vi "pruebas con Alarm Log.vi"() -> ()   [LabVIEW 2018]
panel:
  out "Array":i16[][](array[numeric])
  in  "Descending (F)":bool
  out "PQ_Log array out 4":i16[][](array[numeric])
  out "Numeric":i32
  out "PQ_Log array out":i16[](array[numeric])
  out "Boolean array 6":bool[](array[boolean])
  in  "stop":bool
  # "Sag_Indication_Detected"
  # "Swell_Indication_Detected"
  # "Transient_Indication"
  # "200mS_Sag_Swell_Status_Flag"
  # "3s_Sag_Swell_Status_Flag"
  # "10m_Sag_Swell_Status_Flag"
  # "2h_Sag_Swell_Status_Flag"
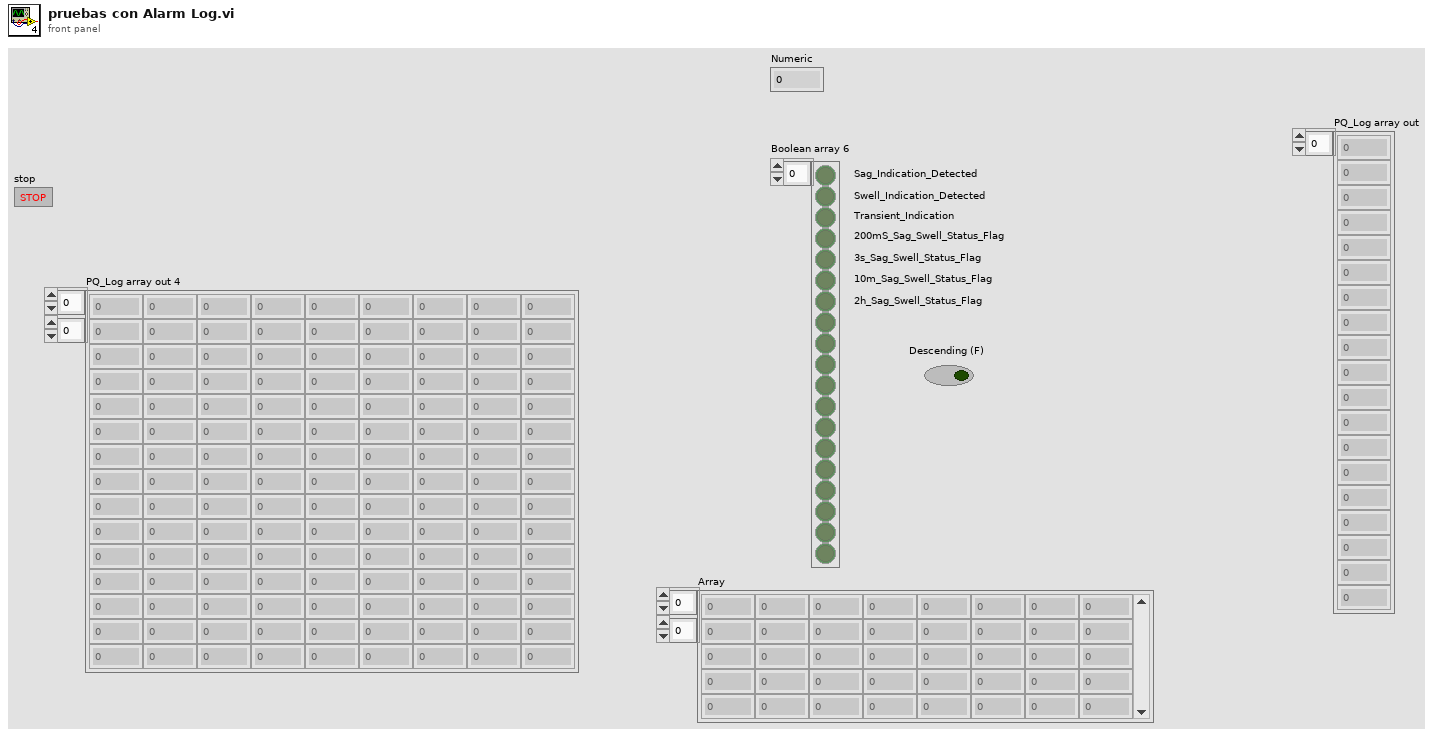
[diagram p1: front panel]
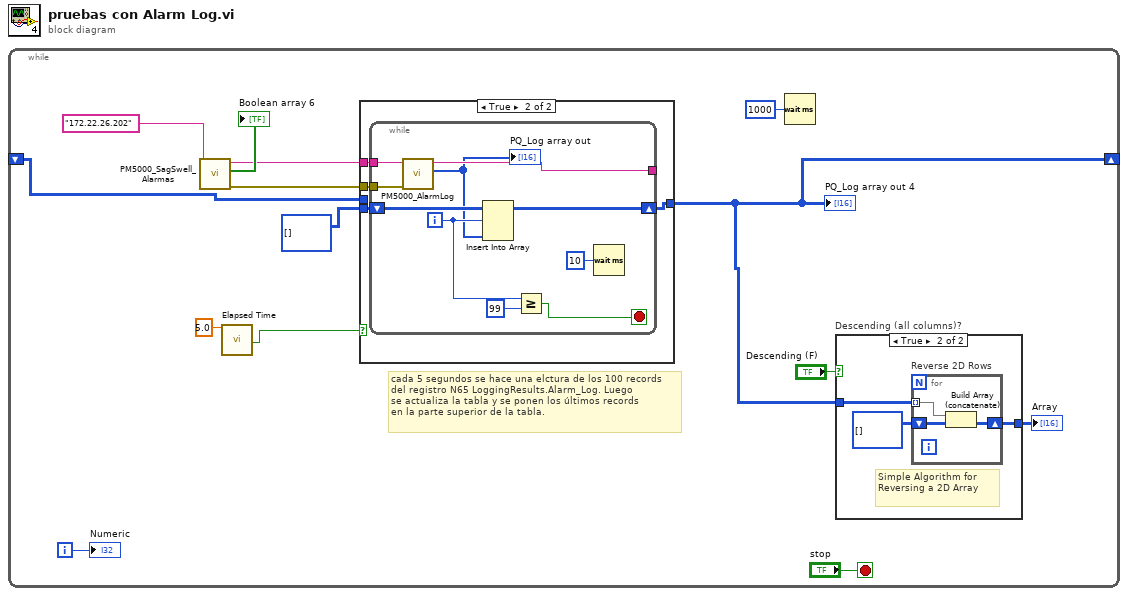
[diagram p0: block diagram]
diagram:
  n1 = while {
    shift-right: [w2] -> _
    shift-left: _ -> [w4]
    i -> [w8]
    stop <- "stop" stop-if-true
    # "cada 5 segundos se hace una elctura de los 100 records\ndel registro N65 LoggingResults.Alarm_Log. Luego\nse actualiza la tabla y se ponen los últimos records \nen la parte superior de la tabla."
    n2 = call "PM5000_SagSwell_Alarmas.vi"("Network Path"="172.22.26.202") -> ("error out"=w9:errorcluster, "PQ_Alarmas"=→"Boolean array 6":bool[], "Network Path out"=w10:string)  [unwired: 8 in]
    n3 = call "Elapsed Time"("Time Target (s)"=5.0) -> ("Time has Elapsed"=w5:bool)  [unwired: 11 in, 7 out]
    n4 = case shown="True" w5 {
      tunnel: w10 -> [_ w26]
      tunnel: w9 -> [_ w25]
      tunnel: i16[][] [] -> [_ w24]
      tunnel: [w22 w23] -> w2
      tunnel: w4 -> [w22 _]
      frame False {
      }
      frame True {
        n5 = while {
          tunnel: w26 -> [w36]
          tunnel: w25 -> [w35]
          tunnel: [w34] -> _
          shift-right: [w32] -> w23
          shift-left: w24 -> [w33]
          i -> [w31]
          stop <- w29 stop-if-true
          n6 = call "PM5000_AlarmLog.vi"("error in"=w35, "Network Path"=w36) -> ("Alarm Log"=w28:i16[], "Network Path out"=w34:string)  [unwired: 7 in, 1 out]
          "PQ_Log array out" <- w28
          n7 = Insert Into Array(array=w33, index (row)=w31, new element=w28) -> (w32:i16[][])  [unwired: 1 in]
          n8 = Greater Or Equal?(x=w31, y=99) -> (x >= y?=w29:bool)
          n9 = Wait (ms)(milliseconds to wait=u32 10) -> ()  [unwired: 1 out]
        }
      }
    }
    "PQ_Log array out 4" <- w2
    n10 = Wait (ms)(milliseconds to wait=u32 1000) -> ()  [unwired: 1 out]
    n11 = case "Descending (all columns)?" shown="True" "Descending (F)" {
      tunnel: w2 -> [w15 w17]
      tunnel: [w15 w16] -> w1
      frame False {
      }
      frame True {
        # "Simple Algorithm for Reversing a 2D Array"
        n12 = for "Reverse 2D Rows" {
          tunnel: w17 -> [w21] mode=indexing
          shift-right: [w19] -> w16
          shift-left: i16[][] [] -> [w20]
          n13 = Build Array (concatenate)(w21, w20) -> (w19:i16[][])
        }
      }
    }
    "Array" <- w1
    "Numeric" <- w8
  }
